vi "Which_Trav_Setup.vi"(1 "Extra Command String":string) -> (0 "Traverse Setups":string[](array[string]))   [LabVIEW 2013]
uses:
  Globals/Extra_Commands_Global.vi
  Globals/Trav_pos_global.vi
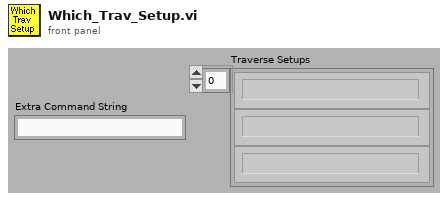
[diagram p1: front panel]
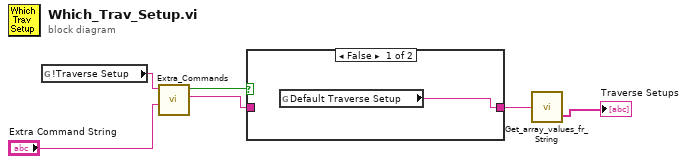
[diagram p0: block diagram]
diagram:
  n1 = global read "Extra_Commands_Global.vi" "!Traverse Setup"() -> (w4:string)
  n2 = call "Extra_Commands.vi"("String to Search"="Extra Command String", "Command"=w4) -> ("String Value"=w6:string, "Command Found"=w5:bool)  [unwired: 1 in, 3 out]
  n3 = case shown="False" w5 {
    tunnel: [w7 w8] -> w2
    tunnel: w6 -> [_ w8]
    frame False {
      n4 = global read "Trav_pos_global.vi" "Default Traverse Setup"() -> (w7:string)
    }
    frame True {
    }
  }
  n5 = call "Get_array_values_fr_String.vi"("String Value"=w2) -> ("String array"=→"Traverse Setups":string[])  [unwired: 1 out]
